vi "MuxReset.vi"(8 "error in (no error)":errorcluster, 11 "KE3700A in":refnum<class "KE3706A.lvclass">) -> (0 "error out":errorcluster, 3 "KE3700A out":refnum<class "KE3706A.lvclass">)   [LabVIEW 2018, in "KE3706A.lvclass"]
uses:
  KE3706A.lvclass
  additional LV libraries/Keithley 3706/Keithley 3700 Series.lvlib
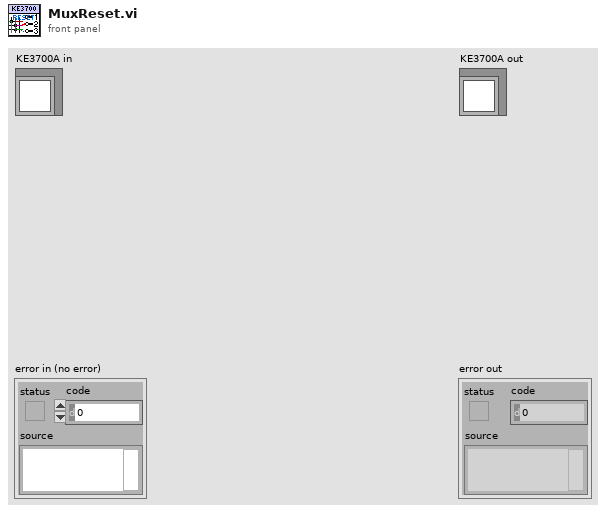
[diagram p1: front panel]
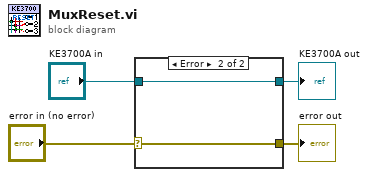
[diagram p0: block diagram]
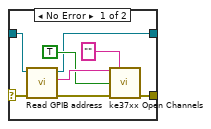
[diagram p2: hidden frame]
diagram:
  n1 = case shown="Error" "error in (no error)" {
    selector: "error in (no error)" -> [w11 w13]
    tunnel: "KE3700A in" -> [w12 w14]
    tunnel: [w6 w14] -> w2
    tunnel: [w5 w13] -> w1
    frame No Error {
      n2 = call-dynamic "Read GPIB address.vi"("error in (no error)"=w11, "InstControl in"=w12) -> ("error out"=w7:errorcluster, "GPIB address"=w10:string, "InstControl out"=w6:refnum<class "KE3706A.lvclass">)  [unwired: 7 in]
      n3 = call "ke37xx Open Channels.vi"("VISA Resource Name"=w10, "Channel List"="", "Open All (False)"=TRUE, "error in (no error)"=w7) -> ("error out"=w5:errorcluster)  [unwired: 10 in, 1 out]
    }
    frame Error {
    }
  }
  "error out" <- w1
  "KE3700A out" <- w2
